vi "Get Key Value Changes.vi"(8 "error in (no error)":errorcluster, 10 "Carya Config (org)":refnum<class "Carya Config.lvclass">, 11 "Carya Config (new)":refnum<class "Carya Config.lvclass">) -> (0 "error out":errorcluster, 1 "Key names":string[](array[string]), 2 "Section names":string[](array[string]), 3 "Carya Config (new)":refnum<class "Carya Config.lvclass">, 4 "Values":string[](array[string]))   [LabVIEW 2013, in "Carya Config.lvclass"]
doc: "Copyright 2018, Carya Automatisering, Wiebe Walstra."
uses:
  Carya Config.lvclass
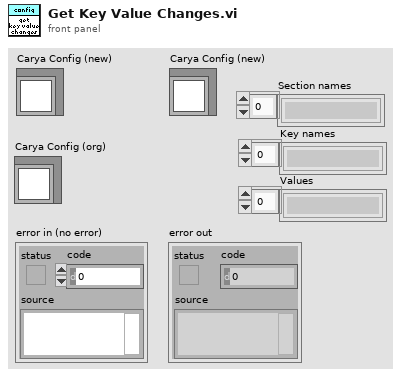
[diagram p1: front panel]
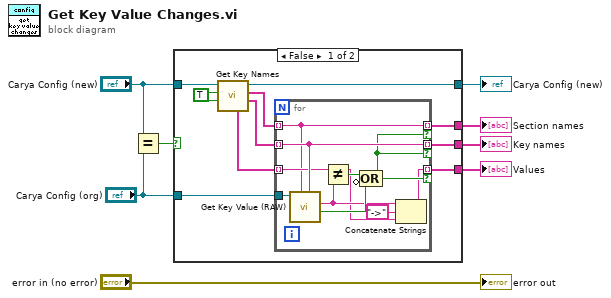
[diagram p0: block diagram]
diagram:
  n1 = Equal?(x="Carya Config (new)", y="Carya Config (org)") -> (x = y?=w1:bool)
  n2 = case shown="False" w1 {
    tunnel: "Carya Config (org)" -> [w11 _]
    tunnel: "Carya Config (new)" -> [w15 w29]
    tunnel: [w9 w29] -> w5
    tunnel: [w14 _] -> w4
    tunnel: [w13 _] -> w3
    tunnel: [w12 _] -> w2
    frame False {
      w18 = TRUE ("Use Section Regex? [F]")
      n3 = call-dynamic "Get Key Names.vi"("Use Key Regex? [F]"=w18, "Use Section Regex? [F]"=w18, "Carya Config in"=w15) -> ("Key names"=w16:string[], "Section names"=w17:string[], "Carya Config out"=w9:refnum<class "Carya Config.lvclass">, "Context (concatenated)"=w10:string[])  [unwired: 4 in, 1 out]
      n4 = for {
        tunnel: w17 -> [w19] mode=indexing
        tunnel: w16 -> [w25] mode=indexing
        tunnel: w11 -> [w28]
        tunnel: [w19] -> w14 mode=indexing if=w24
        tunnel: [w23] -> w12 mode=indexing if=w24
        tunnel: [w25] -> w13 mode=indexing if=w24
        tunnel: w10 -> [w20] mode=indexing
        n5 = call-dynamic "Get Key Value (RAW).vi"("Key name"=w25, "Section name"=w19, "Carya Config in"=w28) -> ("Found?"=w26:bool, "Value"=w21:string)  [unwired: 5 in, 2 out]
        n6 = Not Equal?(x=w20, y=w21) -> (x != y?=w27:bool)
        n7 = Compound Arithmetic op=OR(w27, invert w26) -> (w24:bool)
        n8 = Concatenate Strings(w21, "->" ("string"), w20) -> (w23:string)
      }
    }
    frame True {
    }
  }
  "Carya Config (new)" <- w5
  "Section names" <- w4
  "Key names" <- w3
  "Values" <- w2
  "error out" <- "error in (no error)"
